vi "rqcAlice FPGA.vi"() -> ()   [LabVIEW 2018]
uses:
  Alice/Custom Controls/Main State Machine/rqcAlice DAC Clock Positions.ctl
  Alice/Custom Controls/Phase Modulator/rqcAlice Mod.Config.ctl
  Shared/Shared FPGA Lib/Shared Logic/Custom Controls/rqc Random Generator.parameters.ctl
  Shared/Shared FPGA Lib/Shared Logic/Custom Controls/rqc Random Generator.value type.ctl
  <vilib>/Platform/TimedLoop/XDataNode/timing_clust.ctl
  <vilib>/Platform/TimedLoop/XDataNode/nitl_modes.ctl
  <vilib>/Platform/TimedLoop/XDataNode/wakeup.ctl
  <vilib>/rvi/Emulation/niFpgaSctlEmulationGetInTimedLoop.vi
  <vilib>/rvi/Emulation/niFpgaEmulationReportErrorSimple.vi
  <vilib>/rvi/Emulation/niFpgaGetClockAttributes.vi
  <vilib>/rvi/Emulation/niFpgaCriticalErrorInLSC.vi
  <vilib>/rvi/eio/common/nirviEmuTemplateMethod_errors.vi
  <vilib>/rvi/Emulation/niFpgaEmulationIsFPGAContextNoSignature.vi
  <vilib>/rvi/DataTransferAndStorage/Container/Common/niFpgaContainerGetUniqueNameForEmu.vi
  <vilib>/rvi/eio/common/nirviEmuReportErrorAndStop.vi
  <vilib>/rvi/Emulation/niFpgaProcessEmulError.vi
  <vilib>/rvi/Memory/Memory_Emulation/niFpgaMemoryEmulationCacheClearOnFirstRun.vi
  <vilib>/rvi/Memory/Memory_Emulation/nirvimemoryEmulationManagerCache_MakeExclusive.vi
  <vilib>/rvi/Memory/Memory_Emulation/niFpgaMemoryEmulationValidateCache.vi
  <vilib>/rvi/Memory/Memory_Emulation/nirvimemoryEmulationManagerCache_InsertValue.vi
  <vilib>/Utility/error.llb/Clear Errors.vi
  <vilib>/rvi/Memory/Memory_Emulation/nirvimemoryEmulationManagerCache_ReleaseExclusive.vi
  <vilib>/rvi/Memory/Memory_Emulation/nirvimemoryEmulationManagerCache_GetValue.vi
  <vilib>/rvi/Memory/Memory_Emulation/nirvimemoryEmulationManagerCache_SetValue.vi
  Shared/Shared FPGA Lib/Shared Logic/FIFO/FIFO.write/rqc FIFO Write (U8).vi
  <vilib>/rvi/DataTransferAndStorage/Container/Common/niFpgaContainerSetEmuInfo.vi
  <vilib>/Platform/TimedLoop/XDataNode/XDataNode.xnode
  <vilib>/eio/EIONode/EIONode.xnode
  <vilib>/rvi/DataTransferAndStorage/Container/XNode/niFpgaContainer.xnode
  <vilib>/rvi/DataTransferAndStorage/Handshake/Emulation/niFpgaHandshakeEmulation.vi
  <vilib>/rvi/DataTransferAndStorage/Register/Emulation/niFpgaRegisterEmulation.vi
  <vilib>/rvi/LocalResourceManager/LocalResourceManager.xnode
  <vilib>/Platform/TimedLoop/XDataNode/XDNodeRunTimeDep.lvlib
panel:
  in  "SD/Coax Select":bool
  in  "rndGen.initial seed":u32=4294967295 caption="seed"
  in  "rndGen.parameters":T1={"value type"=enum."constant", "constant"=0, "num of levels"=0, "levels values"=[0, 0, 0, 0]}
  in  "rndGen.reset":bool
  in  "SPI.write":bool
  in  "SPI.data":u32
  out "pm.FIFO timeout":bool
  in  "modulator.config":T3
  in  "DAC.clock positions":T4=[20, 40]
  in  "reset":bool
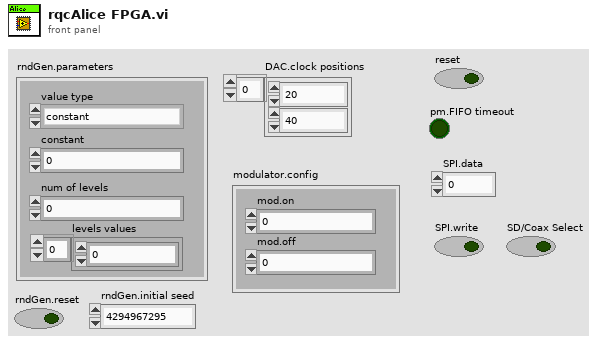
[diagram p1: front panel]
types:
  T1 = typedef "rqc Random Generator.parameters.ctl" = cluster{"value type":T2, "constant":u16, "num of levels":u16, "levels values":u16[]}
  T2 = typedef "rqc Random Generator.value type.ctl" = enum16{"random value", "constant"}
  T3 = typedef "rqcAlice Mod.Config.ctl" = cluster{"mod.on":u8, "mod.off":u8}
  T4 = typedef "rqcAlice DAC Clock Positions.ctl" = u8[]
  T5 = typedef "XDNodeRunTimeDep.lvlib/timing_clust.ctl" = cluster{"Expected End [f-1]":u64, "Actual End [f-1]":u64, "Finished Late? [f-1]":bool, "Expected End [i-1]":u64, "Actual End [i-1]":u64, "Finished Late? [i-1]":bool, "Expected Start [i]":u64, "Actual Start [i]":u64, "Expected Start [f]":u64, "Actual Start [f]":u64, "Source Name":string, "Structure Name":string, "Period":i64, "Deadline":i64, "Offset":i64, "Start":i64, "Priority":i32, "Timeout":i32, "Mode":T6, "Wakeup Reason":T7, "Error":errorcluster, "Source Type":string, "Secondary Source Type":string, "Global End Time":u64, "Global Start Time":u64, "Frame Duration":u64, "Iteration Duration":u64, "Assigned CPU":i32, "I/O Scan Engine Mode":u32}
  T6 = typedef "XDNodeRunTimeDep.lvlib/nitl_modes.ctl" = enum32{"No Change", "Process missed periods, maintain original phase", "Discard missed periods, maintain original phase", "Process missed periods, ignore original phase", "Discard missed periods, ignore original phase"}
  T7 = typedef "XDNodeRunTimeDep.lvlib/wakeup.ctl" = enum32{"Normal", "Aborted", "Asynchronous wakeup", "Timing source error", "Timed loop error", "Timeout"}
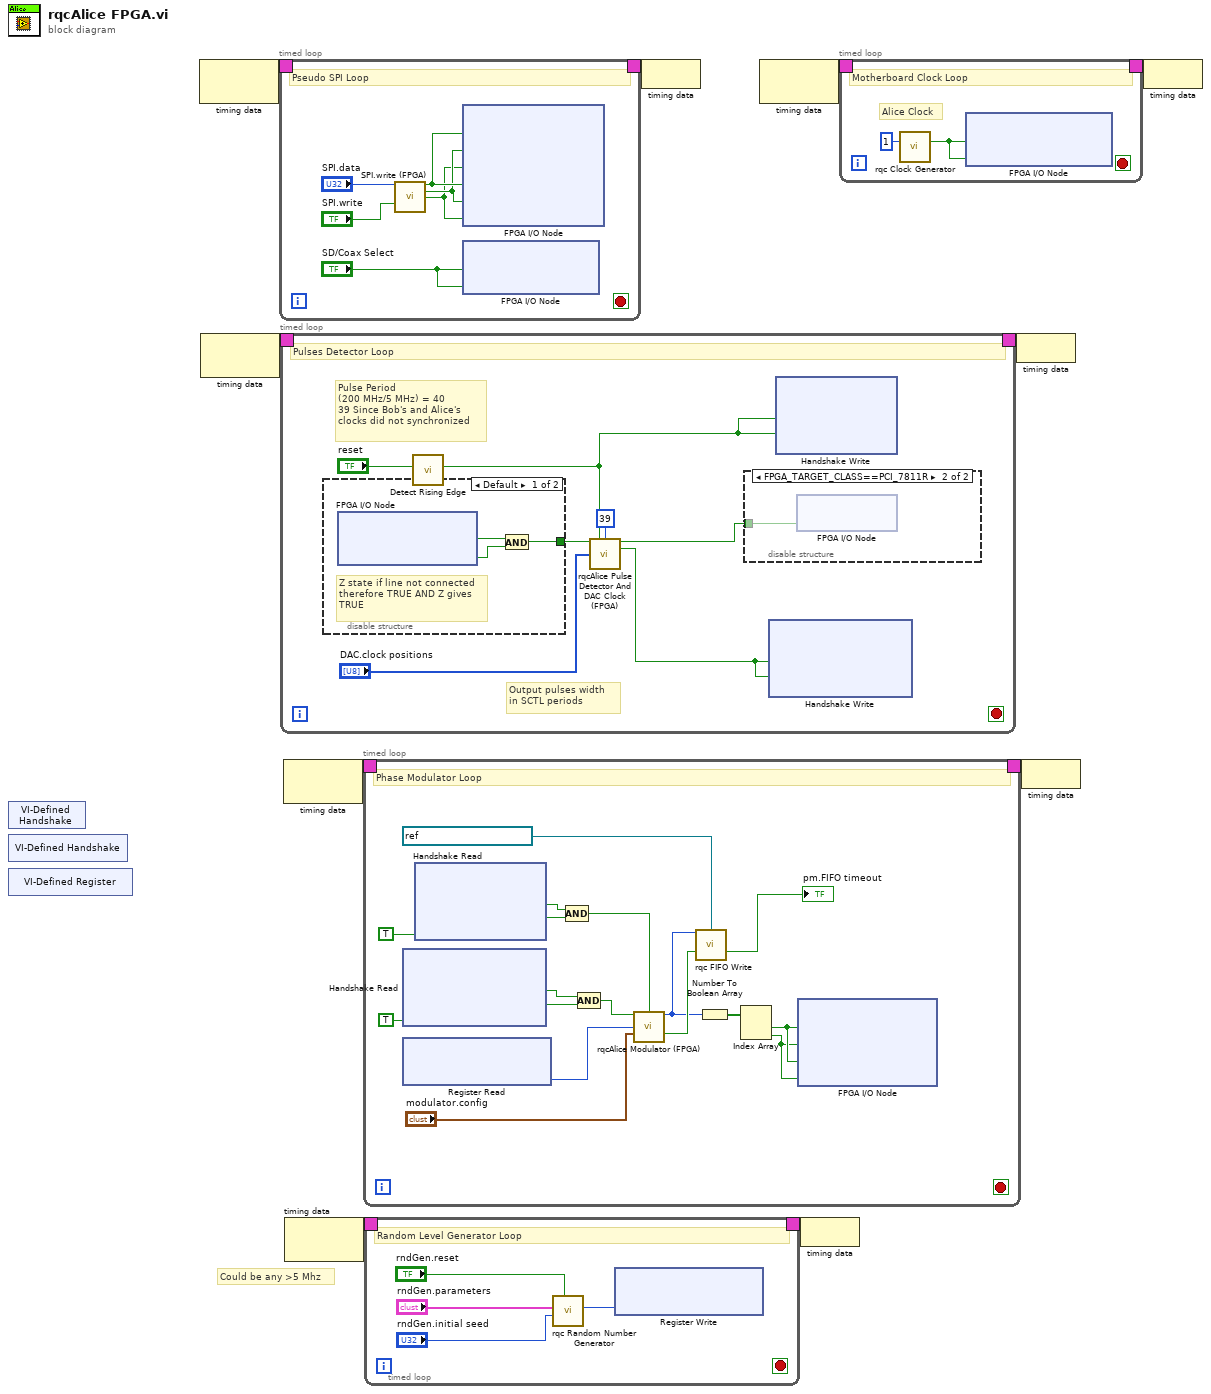
[diagram p0: block diagram]
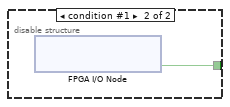
[diagram p2: hidden frame]
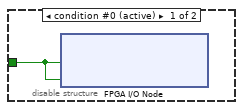
[diagram p3: hidden frame]
diagram:
  # "Could be any >5 Mhz"
  n1 = xnode "VI-Defined Handshake"() -> ()  [unwired: 1 out]
  n2 = xnode "VI-Defined Handshake"() -> ()  [unwired: 1 out]
  n3 = xnode "VI-Defined Register"() -> ()  [unwired: 1 out]
  n4 = node-c288() -> (w6:T5)  [unwired: 1 in]
  n5 = node-c288() -> (w10:T5)  [unwired: 1 in]
  n6 = timed-loop {
    timing: w6 -> [_]
    timing-out: [_] -> w5
    stop <- _ stop-if-true
    # "Pseudo SPI Loop"
    n7 = call "SPI.write (FPGA).vi"("data in"="SPI.data", "write"="SPI.write") -> ("data"=w14:bool, "we"=w13:bool, "clk"=w12:bool)  [unwired: 11 in]
    n8 = xnode "FPGA I/O Node"("SPI/DATA (service)"=w14, "SPI/EN (service)"=w13, "SPI/CLK (service)"=w12, "SPI/Data"=w14, "SPI/EN"=w13, "SPI/CLK"=w12) -> ()  [unwired: 6 in, 6 out]
    n9 = xnode "FPGA I/O Node"("SD/Coax"="SD/Coax Select", "SD/Coax (service)"="SD/Coax Select") -> ()  [unwired: 2 in, 2 out]
  }
  n10 = timed-loop {
    timing: w10 -> [_]
    timing-out: [_] -> w9
    stop <- _ stop-if-true
    # "Output pulses width \nin SCTL periods"
    # "Pulse Period \n(200 MHz/5 MHz) = 40\n39 Since Bob's and Alice's \nclocks did not synchronized"
    # "Pulses Detector Loop"
    n11 = disable-structure shown="Default" {
      disable-tunnel: [w27 w29] -> w20
      frame condition #0 (active) {
        # "Z state if line not connected\ntherefore TRUE AND Z gives\nTRUE"
        n12 = xnode "FPGA I/O Node"() -> ("DelayLineSignal"=w28:bool, "DelayLine(Service)"=w26:bool)  [unwired: 2 in, 2 out]
        n13 = And(x=w28, y=w26) -> (x .and. y?=w27:bool)
      }
      frame condition #1 {
        n14 = xnode "FPGA I/O Node"() -> ("DelayLineSignal"=w29:bool)  [unwired: 1 in, 1 out]
      }
    }
    n15 = call <vilib>:"Detect Rising Edge.vi"("signal"="reset") -> ("edge detected"=w21:bool)  [unwired: 10 in]
    n16 = call "rqcAlice Pulse Detector And DAC Clock (FPGA).vi"("delay line signal"=w20, "reset"=w21, "period"=u8 39 ("main.period"), "DAC clock positions"="DAC.clock positions") -> ("DAC clock"=w19:bool, "pusle arrived"=w23:bool)  [unwired: 10 in]
    n17 = disable-structure shown="FPGA_TARGET_CLASS==PCI_7811R" {
      disable-tunnel: w19 -> [w30 w31]
      frame condition #0 (active) {
        n18 = xnode "FPGA I/O Node"("DAC/clock"=w30, "DAC/clock (service)"=w30) -> ()  [unwired: 2 in, 2 out]
      }
      frame condition #1 {
        n19 = xnode "FPGA I/O Node"("DAC/clock"=w31) -> ()  [unwired: 1 in, 1 out]
      }
    }
    n20 = xnode ("Handshake Write")("Data"=w23, "Input Valid"=w23) -> ()  [unwired: 1 in, 2 out]
    n21 = xnode ("Handshake Write")("Data"=w21, "Input Valid"=w21) -> ()  [unwired: 1 in, 2 out]
  }
  n22 = node-c288() -> (w8:T5)  [unwired: 1 in]
  n23 = node-c288() -> (w2:T5)  [unwired: 1 in]
  n24 = timed-loop {
    timing: w8 -> [_]
    timing-out: [_] -> w7
    stop <- _ stop-if-true
    # "Phase Modulator Loop"
    n25 = xnode ("Handshake Read")("Ready for Output"=TRUE) -> ("Data"=w45:bool, "Output Valid"=w44:bool)  [unwired: 1 in, 1 out]
    n26 = xnode ("Register Read")() -> ("Data"=w46:u8)  [unwired: 1 in, 1 out]
    n27 = xnode ("Handshake Read")("Ready for Output"=TRUE) -> ("Data"=w40:bool, "Output Valid"=w39:bool)  [unwired: 1 in, 1 out]
    n28 = Compound Arithmetic op=AND(w40, w39) -> (w38:bool)
    n29 = Compound Arithmetic op=AND(w45, w44) -> (w42:bool)
    n30 = call "rqcAlice Modulator (FPGA).vi"("pulse arrived"=w42, "reset"=w38, "DAC random level"=w46, "rqcAlice PM.config"="modulator.config") -> ("DAC level"=w37:u8, "DAC value changed"=w49:bool)  [unwired: 10 in]
    n31 = call-poly "rqc FIFO Write.vi"("Element"=w37, "FIFO"=refnum<k21> "FIFO PM DAC Level" ("FIFO PM DAC Level"), "data valid"=w49) -> ("Timed Out?"=→"pm.FIFO timeout":bool)  [unwired: 12 in]
    n32 = Number To Boolean Array(number=w37) -> (Boolean array=w36:bool[])
    n33 = Index Array(array=w36) -> (element #1=w35:bool, element #2=w34:bool)  [unwired: 2 in]
    n34 = xnode "FPGA I/O Node"("DAC/bit2"=w35, "DAC/bit3"=w34, "DAC/bit2 (service)"=w35, "DAC/bit3 (service)"=w34) -> ()  [unwired: 4 in, 4 out]
  }
  n35 = timed-loop {
    timing: w2 -> [_]
    timing-out: [_] -> w1
    stop <- _ stop-if-true
    # "Random Level Generator Loop"
    n36 = call "rqc Random Number Generator.vi"("reset"="rndGen.reset", "initial seed"="rndGen.initial seed", "rndGen.parameters"="rndGen.parameters") -> ("DAC random level"=w56:u8)  [unwired: 8 in]
    n37 = xnode ("Register Write")("Data"=w56) -> ()  [unwired: 1 in, 1 out]
  }
  n38 = node-c288(w5) -> ()
  n39 = node-c288() -> (w4:T5)  [unwired: 1 in]
  n40 = node-c288(w1) -> ()
  n41 = timed-loop {
    timing: w4 -> [_]
    timing-out: [_] -> w3
    stop <- _ stop-if-true
    # "Alice Clock"
    # "Motherboard Clock Loop"
    n42 = call "rqc Clock Generator.vi"("SCTL clock devider"=u8 1) -> ("clock out"=w59:bool)  [unwired: 14 in]
    n43 = xnode "FPGA I/O Node"("AliceClock"=w59, "AliceClock (service)"=w59) -> ()  [unwired: 2 in, 2 out]
  }
  n44 = node-c288(w9) -> ()
  n45 = node-c288(w7) -> ()
  n46 = node-c288(w3) -> ()
